vi "Disconnect from Slave.vi"(8 "error in":errorcluster, 11 "TCP master in":refnum<class "TCP.lvclass">) -> (0 "error out":errorcluster, 3 "TCP master out":refnum<class "TCP.lvclass">)   [LabVIEW 2021, in "TCP.lvclass"]
doc: "Closes the TCP connection stored in the class."
uses:
  TCP.lvclass
  C:/my_projects/projects/Algorithms/Labview/21/Master CR/Master CR.lvclass
  Master CR.lvclass/Master CR.ctl
  Modbus_v121c/Network Protocol/Network Master/Network Master.lvclass/Network Master.ctl
  Network Protocol/Read Network Protocol.vi
  Modbus_v121c/Network Protocol/Network Master/Network Master.lvclass
  C:/my_projects/projects/Algorithms/Labview/21/Modbus_v121c/Network Protocol/Network Protocol.lvclass
  Modbus_v121c/Transmission Data Unit/Transmission Data Unit.lvclass
  Master CR.lvclass
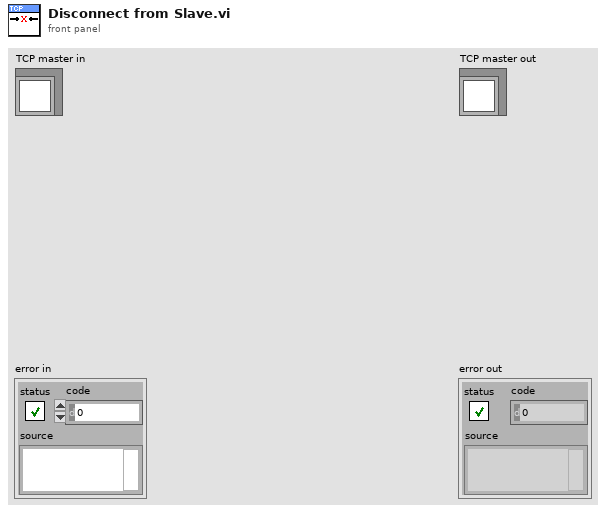
[diagram p1: front panel]
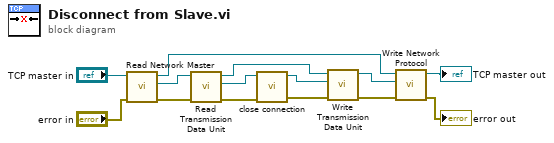
[diagram p0: block diagram]
diagram:
  n1 = call "Read Network Master.vi"("error in (no error)"="error in", "TCP in"="TCP master in") -> ("error out"=w10:errorcluster, "Network Master"=w14:refnum<class "Network Master.lvclass">, "TCP out"=w8:refnum<class "TCP.lvclass">)  [unwired: 7 in]
  n2 = call "Read Transmission Data Unit.vi"("error in (no error)"=w10, "Network Master in"=w14) -> ("error out"=w5:errorcluster, "Transmission Data Unit"=w13:refnum<class "Transmission Data Unit.lvclass">, "Network Master out"=w9:refnum<class "Network Master.lvclass">)  [unwired: 7 in]
  n3 = call-dynamic "close connection.vi"("error in"=w5, "transmission data unit in"=w13) -> ("error out"=w11:errorcluster, "transmission data unit out"=w12:refnum<class "Transmission Data Unit.lvclass">)  [unwired: 8 in]
  n4 = call "Write Transmission Data Unit.vi"("error in (no error)"=w11, "Transmission Data Unit"=w12, "Network Master in"=w9) -> ("error out"=w6:errorcluster, "Network Master out"=w7:refnum<class "Network Master.lvclass">)  [unwired: 7 in]
  n5 = call "Write Network Protocol.vi"("error in (no error)"=w6, "Network Protocol"=w7, "Master CR in"=w8) -> ("error out"=→"error out":errorcluster, "Master CR out"=→"TCP master out":refnum<class "TCP.lvclass">)  [unwired: 7 in]
